vi "S2C_UNITHERM_Proc_SendCmd.vi"(8 "Error In":errorcluster, 11 "Q-Ref":refnum<queue>) -> (0 "Error Out":errorcluster, 3 "Command":string)   [LabVIEW 2024]
uses:
  S2C_UNITHERM_Proc_Globals.vi
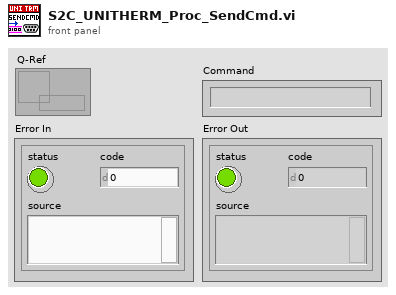
[diagram p1: front panel]
types:
  T1 = cluster{"Caller-Q":refnum<queue>, "Command":string, "Return":string, "Data":variant, "Timeout":dbl}
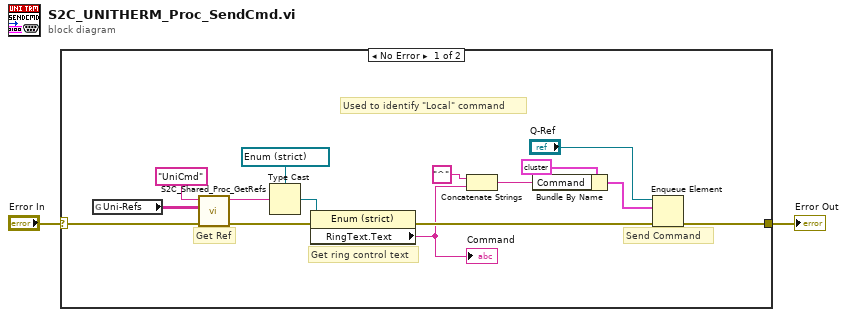
[diagram p0: block diagram]
diagram:
  n1 = case shown="No Error" "Error In" {
    selector: "Error In" -> [w8 w18]
    tunnel: [w3 w18] -> w1
    frame No Error {
      # "Get ring control text"
      # "Get Ref"
      # "Used to identify \"Local\" command"
      # "Send Command"
      n2 = global read "S2C_UNITHERM_Proc_Globals.vi" "Uni-Refs"() -> (w5:string[][])
      n3 = call "S2C_Shared_Proc_GetRefs.vi"("Error In"=w8, "Refs"=w5, "Label"="UniCmd") -> ("Error Out"=w9:errorcluster, "Reference"=w12:string)  [unwired: 7 in]
      n4 = Type Cast(type=refnum<vi> refnum ("Enum"), x=w12) -> (*(type *) &x=w10:refnum<vi>)
      n5 = property class="Enum (strict)"(reference=w10, error in=w9) -> (error out=w6:errorcluster, "RingText.Text"=w4:string)  [unwired: 1 out]
      "Command" <- w4
      n6 = Concatenate Strings("^" ("string"), w4) -> (w13:string)
      n7 = Bundle By Name(cluster=T1 {"Caller-Q"=refnum, "Command"="", "Return"="Local", "Data"=variant, "Timeout"=10.0} ("element"), "Command"=w13) -> (w15:T1)
      n8 = Enqueue Element(queue="Q-Ref", element=w15, error in (no error)=w6) -> (error out=w3:errorcluster)  [unwired: 1 in, 2 out]
    }
    frame Error {
    }
  }
  "Error Out" <- w1
